vi "ResetLift.vi"() -> ()   [LabVIEW 2016, in "LEGO-PMR.lvrbt"]
uses:
  LEGO-PMR.lvrbt
  <vilib>/NXT/Block Support/NXT_ButtonSelector.ctl
  <vilib>/NXT/Dual Mode Library/Display/drawText_Center.vi
  <vilib>/NXT/Dual Mode Library/Sensors/readNXTButton.vi
panel:
  out "Exit Condition":bool
  out "Arm is Up?":bool
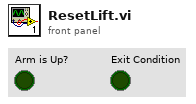
[diagram p1: front panel]
types:
  T1 = typedef "NXT_ButtonSelector.ctl" = u16
  T2 = typedef "LVHSConnector.ctl" = refnum<class "BrickReference.lvclass">
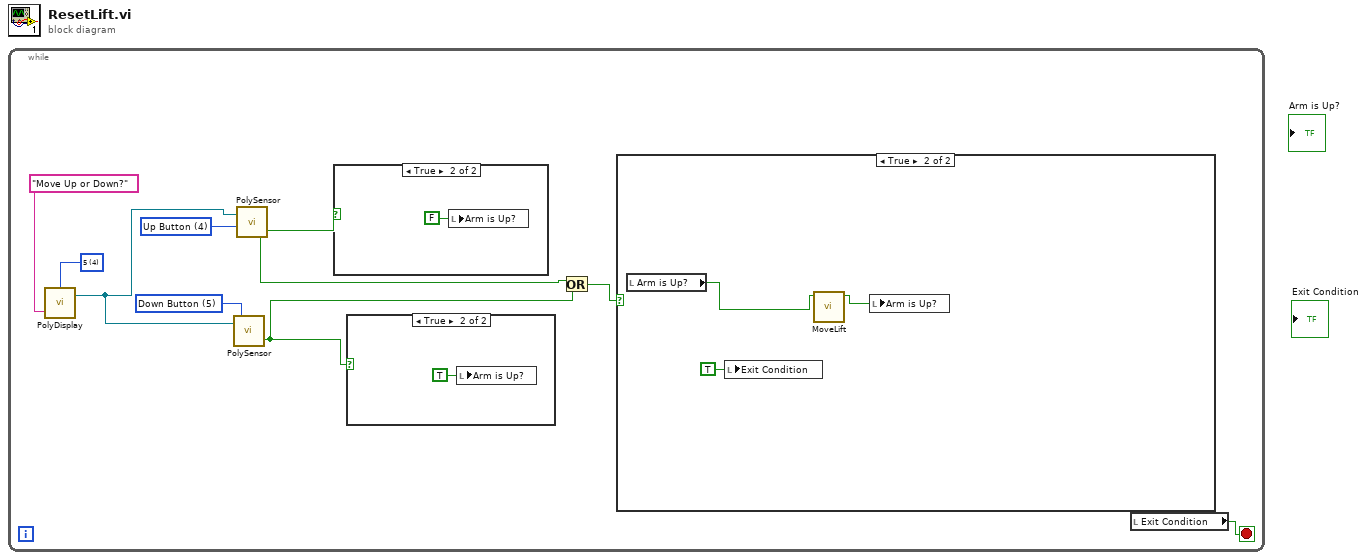
[diagram p0: block diagram]
diagram:
  n1 = while {
    stop <- w1 stop-if-true
    w6 = T1 5 items=["Enter button"=3, "Left button"=2, "Right button"=1, "Up Button"=4, "Down Button"=5] ("Button (Enter button)")
    w5 = T1 4 items=["Enter button"=3, "Left button"=2, "Right button"=1, "Up Button"=4, "Down Button"=5] ("Button (Enter button)")
    w3 = i16 4 items=["1", "2", "3", "4", "5", "6", "7", "8", "9", "10", "11", "12"] ("Line")
    n2 = call-poly <vilib>:"PolyDisplay.vi"("Text"="Move Up or Down?", "Line"=w3) -> ("NXT/EV3"=w9:T2)  [unwired: 2 in]
    n3 = call-poly <vilib>:"PolySensor.vi"("Button (Enter button)"=w6, "NXT/EV3"=w9) -> ("Yes/No"=w7:bool)  [unwired: 1 in, 1 out]
    n4 = call-poly <vilib>:"PolySensor.vi"("Button (Enter button)"=w5, "NXT/EV3"=w9) -> ("Yes/No"=w8:bool)  [unwired: 1 in, 1 out]
    n5 = case shown="True" w8 {
      frame False {
      }
      frame True {
        n6 = local write "Arm is Up?"(FALSE ("Arm is Up?")) -> ()
      }
    }
    n7 = case shown="True" w7 {
      frame False {
      }
      frame True {
        n8 = local write "Arm is Up?"(TRUE ("Arm is Up?")) -> ()
      }
    }
    n9 = Or(x=w8, y=w7) -> (x .or. y?=w2:bool)
    n10 = case shown="True" w2 {
      frame False {
      }
      frame True {
        n11 = local read "Arm is Up?"() -> (w11:bool)
        n12 = local write "Exit Condition"(TRUE ("Exit Condition")) -> ()
        n13 = call "MoveLift.vi"("Arm is Up?"=w11) -> ("Updated Bool"=w10:bool)  [unwired: 10 in]
        n14 = local write "Arm is Up?"(w10) -> ()
      }
    }
    n15 = local read "Exit Condition"() -> (w1:bool)
  }
